vi "ICRA2024测试椭圆分裂.vi"() -> ()   [LabVIEW 2018]
doc: "Demonstrates the use of the Network Streams functions to send LED status to the myRIO target."
uses:
  <vilib>/vision/Contour.llb/IMAQ Contour Curve Extraction.ctl
  <vilib>/ErrorRing/Error Ring.xnode
  <vilib>/vision/NI_Vision_Development_Module.lvlib
panel:
  in  "Search Rect (entire image)":T1={"Left"=200, "Top"=120, "Right"=2000, "Bottom"=1920, "Rotation"=0.0} {"Rotation" format="%.2f"; "Left" scale=0.0..1024.0; "Right" scale=0.0..1024.0}
  out "长度":dbl
  out "备用的椭圆角度":sgl
  in  "打开轨迹":bool
  out "Image 9":T2(plugin-control)
  in  "Search Direction":T3(ring)
  in  "Contour Selection":T4(ring)
  in  "Number of Erosion":i32=10
  in  "椭圆磁场开关":bool=TRUE
  out "Image 7":T2(plugin-control)
  out "Ellipse":T5 {"Center"."Y" format="%.2f"; "Center"."X" format="%.2f"}
  out "Image 5":T2(plugin-control)
  in  "Contour Points Settings":T6={"Overlay?"=FALSE, "Color"=16711680, "Width"=1, "Maintain Width?"=TRUE}
  in  "Contour Equation Settings":T6={"Overlay?"=TRUE, "Color"=3381759, "Width"=1, "Maintain Width?"=TRUE}
  out "ROI Descriptor Out":T7 {"Contours"."Type" items=["No Selection", "Point", "Line", "Rectangle", "Oval", "Polygon", "Freehand Region", "Annulus", "Unused2", "Unused3", "Broken Line", "Freehand Line", "Rotated Rectangle"]}
  in  "Curve Extraction":T8={"Extraction Mode"=0, "Edge Threshold"=75, "Edge Filter Size"=1, "Min Length"=25, "Search Step Size"=15, "Max Endpoint Gap"=10, "Subpixel"=TRUE} {"Extraction Mode" items=["Normal", "Uniform Regions"]; "Edge Filter Size" items=["Fine", "Normal", "Contour Tracing"]; "Max Endpoint Gap" min=0; "Search Step Size" min=1 max=255 step=1; "Min Length" min=0; "Edge Threshold" min=1 max=350 step=1}
  out "Image 4":T2(plugin-control)
  out "Image":T2(plugin-control)
  in  "Acquisition Control::Acquisition Frame Rate":dbl=19.50304412841797 min=1.4211589097976685 max=44.94382095336914
  out "Stopped":bool
  in  "Stop (F) 2":bool caption="Stop (F)"
  out "Objects 2":T9(array[cluster]) {"Aspect Ratio" format="%.2f"; "Orientation" format="%.2f"; "Area" format="%.2f"; "Object Center"."Y" format="%.2f"; "Object Center"."X" format="%.2f"}
  in  "Settings 2":T10={"Objects"=0, "Threshold"=128, "Reject Border"=FALSE, "Fill Holes"=FALSE, "Min Object Size"=TRUE, "Min Size"=20000, "Max Object Size"=FALSE, "Max Size"=100, "Show Search Area"=FALSE, "Show Center"=TRUE, "Show Bounding Box"=TRUE} {"Objects" items=["Bright Objects", "Dark Objects"]; "Threshold" min=1 max=999999999 step=1; "Max Size" min=1 max=999999999 step=1; "Min Size" min=1 max=999999999 step=1}
  in  "Range 2":cluster{"Lower value":sgl, "Upper value":sgl}={"Lower value"=0.0, "Upper value"=230.0} {"Upper value" format="%.2f"; "Lower value" format="%.2f"}
  in  "Pause":bool
  out "Array":dbl[](array[numeric])
  in  "Parameter Settings":T11(tab)=enum."Ribbon Oscillating Field" caption="Field Types"
  in  "fg":dbl
  in  "pg":dbl
  in  "dg":dbl
  in  "Ag":dbl
  in  "AoOF":dbl
  in  "fo":sgl
  in  "do":sgl
  in  "oo":sgl
  in  "po":sgl
  in  "cc":sgl
  in  "pc":sgl
  in  "wc":sgl
  in  "dc":sgl
  in  "Ac":dbl
  in  "pr":sgl
  in  "Ar":dbl=8.0
  in  "wr":sgl=18.0
  in  "dr":sgl
  in  "Dis phase step":dbl
  in  "Dis phase frequency (Hz)":dbl
  in  "Dis tumbling frequency (Hz)":dbl
  in  "Dis strength(mT)":dbl
  in  "Swa strength (mT)":dbl
  in  "Swa frequency (Hz)":dbl
  in  "Swa pitch angle (deg)":dbl
  in  "Swa direction angle (deg)":dbl
  in  "Swa ratio":dbl=1.0
  in  "Pitch Angle (rotating around Constant, deg)":dbl
  in  "Ratio (A/C)":sgl=4.0
  in  "Direction Angle (deg)":sgl
  in  "Pitch Angle (rotating around Origin, deg)":sgl
  in  "Frequency (Hz)":sgl=10.0
  in  "Strength (mT)":dbl=10.0
  in  "Ar 2":dbl=5.0 caption="Ar"
  in  "ratio":sgl=1.0
  in  "运动方向":sgl
  in  "长轴方向":sgl
  in  "wr  2":sgl=8.0
  in  "速度大小":sgl
  out "Angle":dbl
  out "aspect ratio":dbl
  out "时间":i32
  out "Numeric 5":i32
  in  "Stop":bool
  out "error out":errorcluster
  in  "Target IP Address":string="172.22.11.2"
  # "Overview: Magnetic field calculation, and send parameters to myRIO\nInstructions:\n1. Verify the value of Target IP Address. Set Visa resource name.\n2. Ensure RT Main.vi is already running. \n3. Run this VI. Set parameters of magnetic field."
  # "Strength (mT)"
  # "Pitch Angle (deg)"
  # "Direction Angle (deg)"
  # "Frequency (Hz)"
  # "Strength (mT)"
  # "Oscilation Frequency (Hz)"
  # "Oscilation Angle (deg)"
  # "Pitch Angle (deg)"
  # "Direction Angle (deg)"
  # "Strength (mT)"
  # "Frequency (Hz)"
  # "Pitch Angle (deg)"
  # "Direction Angle (deg)"
  # "Conical Angle (deg)"
  # "Strength (mT)"
  # "Frequency (Hz)"
  # "Pitch Angle (deg)"
  # "Direction Angle (deg)"
  # "Strength (mT)"
  # "Tumbling Frequency (Hz)"
  # "Phase Frequency (Hz)"
  # "Phase Step"
  # "Strength (mT)"
  # "Frequency (Hz)"
  # "Pitch Angle (deg)"
  # "Direction Angle (deg)"
  # "Ratio"
  # "Strength (mT)"
  # "Frequency (Hz)"
  # "Ratio (A/C)"
  # "Direction Angle (deg)"
  # "Pitch Angle (rotating around Origin, deg)"
  # "Pitch Angle (rotating around Constant, deg)"
  # "Strength (mT)"
  # "Frequency (Hz)"
  # "Pitch Angle  (deg)"
  # "longaxis"
  # "Direction Angle (deg)"
  # "ratio (l/s)"
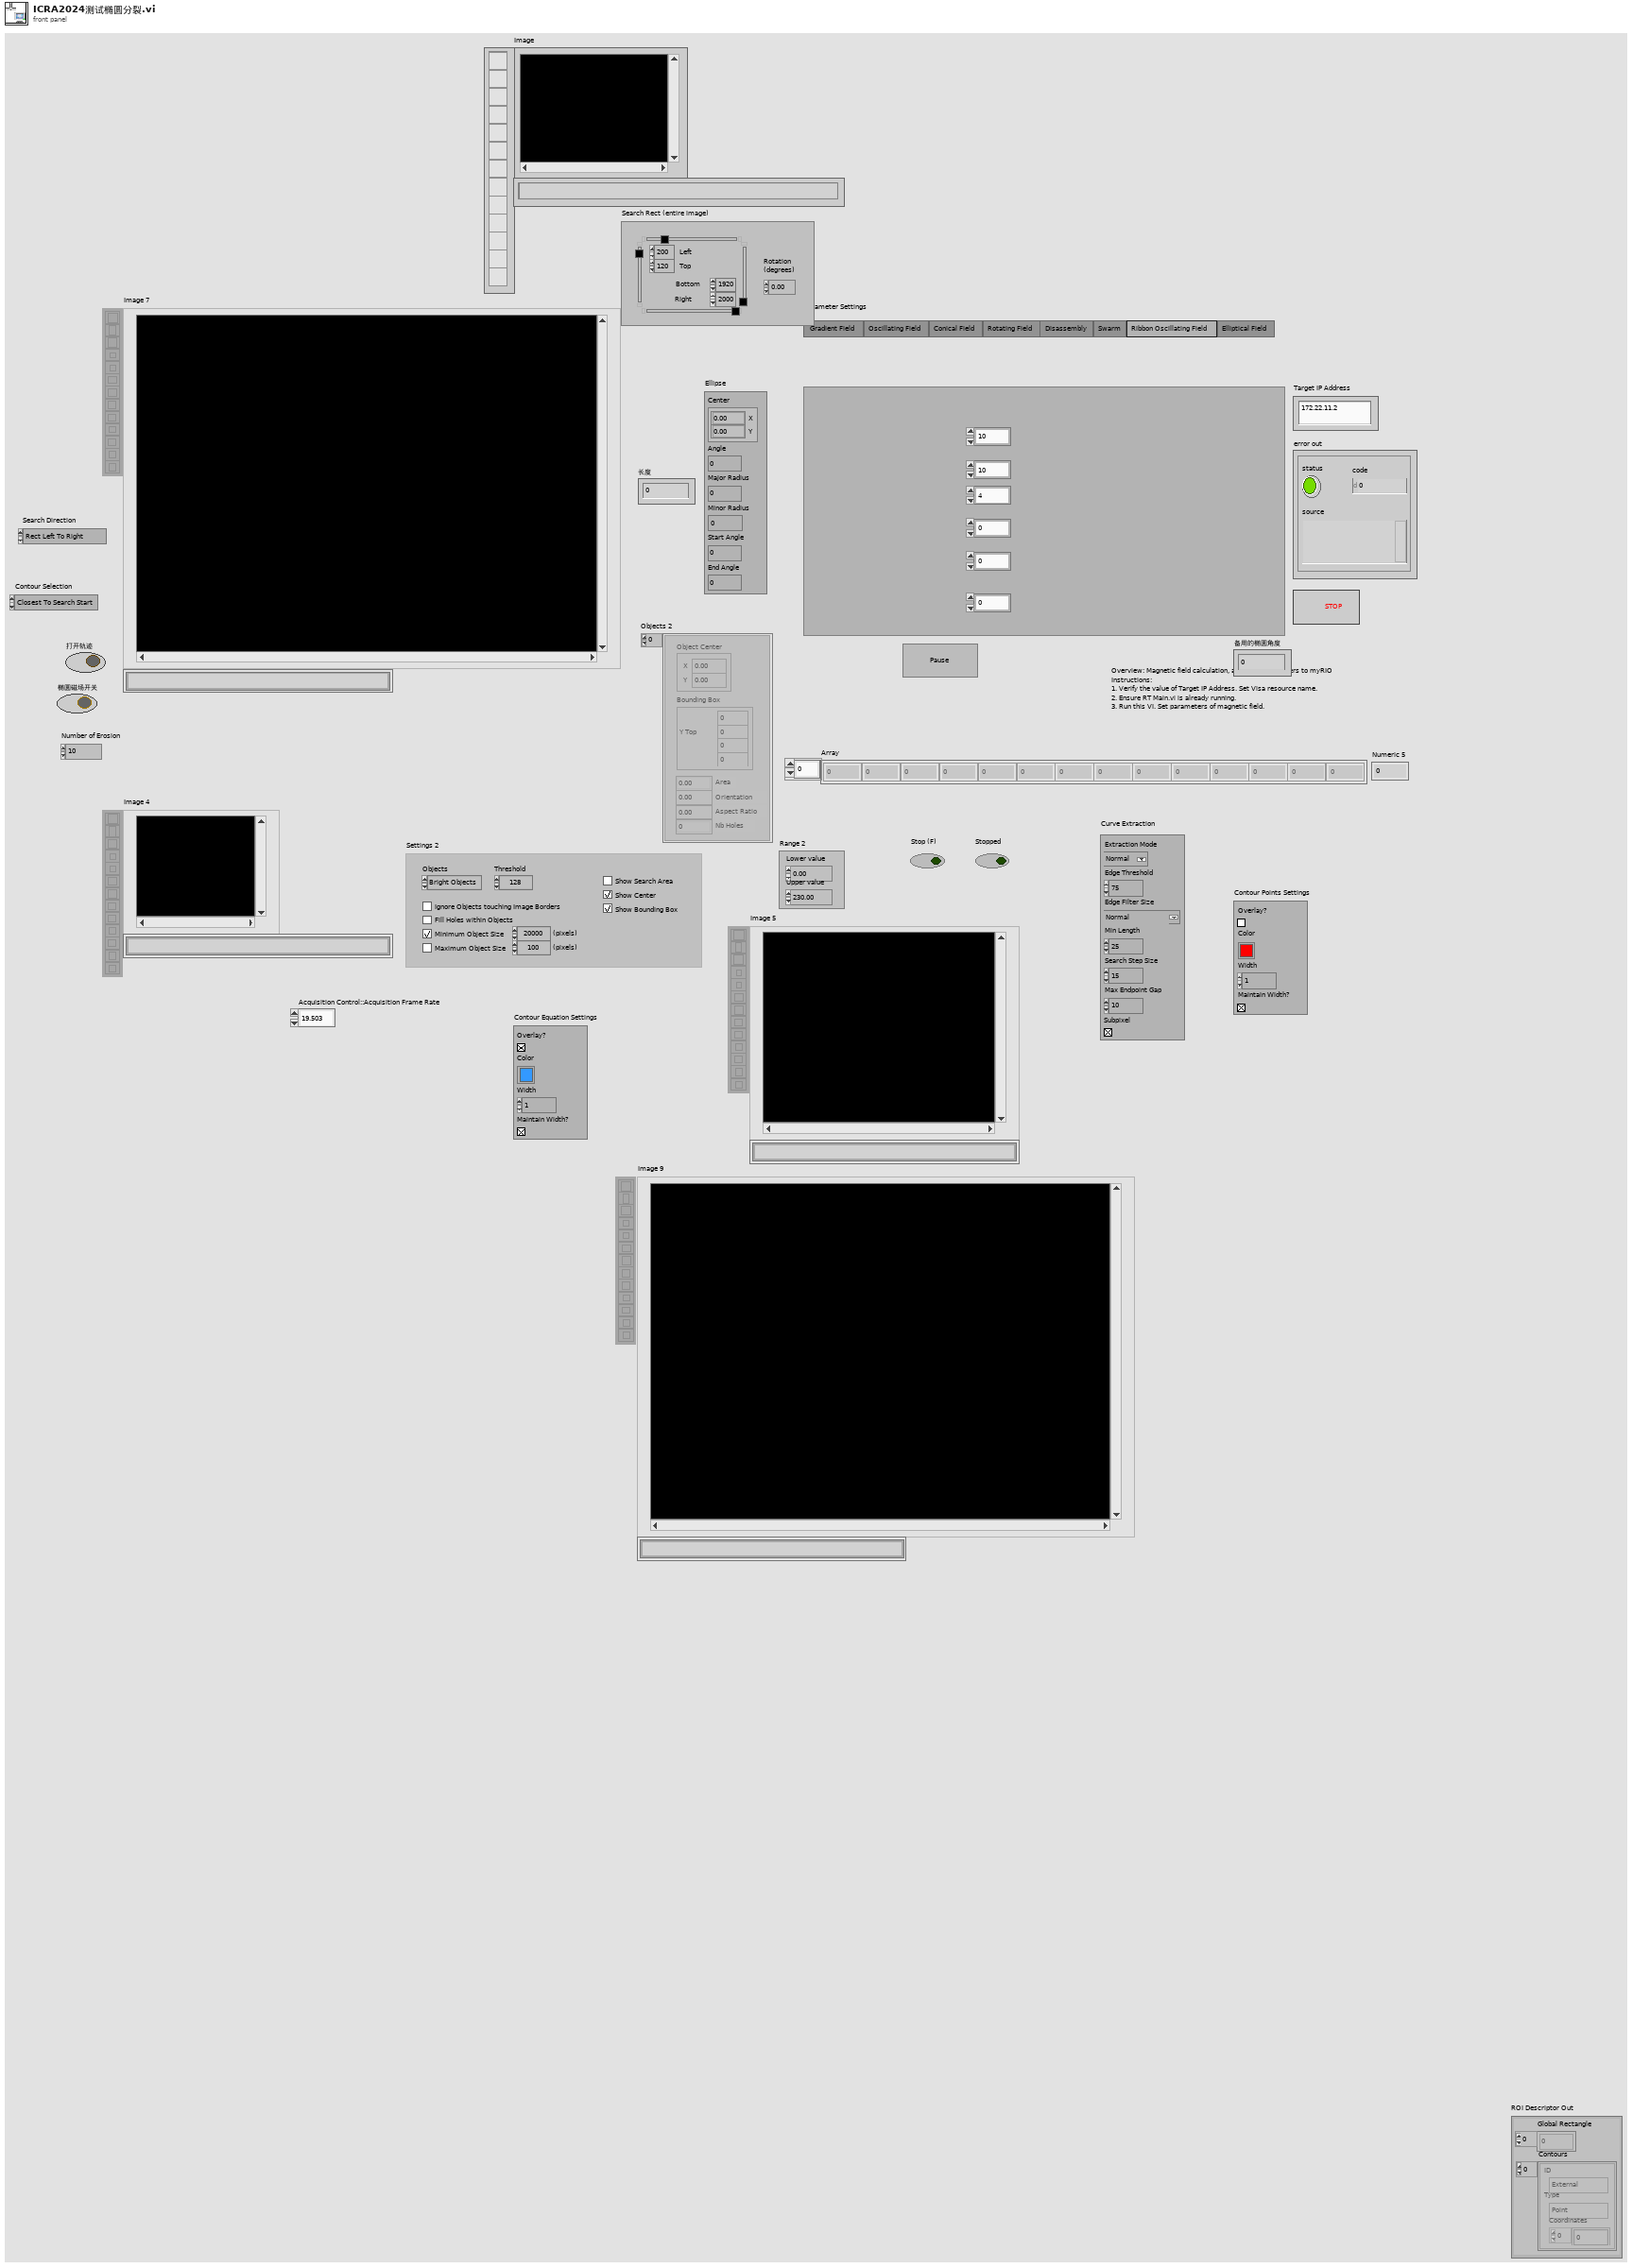
[diagram p1: front panel]
types:
  T1 = typedef "IMAQ Rectangle" = cluster{"Left":i32, "Top":i32, "Right":i32, "Bottom":i32, "Rotation":dbl}
  T2 = typedef "IMAQ Image.ctl" = refnum<image>
  T3 = enum16{"Rect Left To Right", "Rect Right To Left", "Rect Top To Bottom", "Rect Bottom To Top", "Annulus Inner To Outer", "Annulus Outer To Inner", "Annulus Start Angle To End Angle", "Annulus End Angle To Start Angle"}
  T4 = enum16{"Closest To Search Start", "Maximum Length", "Strongest Mean Gradient Change"}
  T5 = cluster{"Center":cluster{"X":sgl, "Y":sgl}, "Angle":dbl, "Major Radius":dbl, "Minor Radius":dbl, "Start Angle":dbl, "End Angle":dbl}
  T6 = cluster{"Overlay?":bool, "Color":u32, "Width":u32, "Maintain Width?":bool}
  T7 = typedef "ROI Descriptor" = cluster{"Global Rectangle":i32[], "Contours":cluster{"ID":enum32{"External", "Internal"}, "Type":u32, "Coordinates":i32[]}[]}
  T8 = typedef "IMAQ Contour Curve Extraction.ctl" = cluster{"Extraction Mode":u32, "Edge Threshold":i32, "Edge Filter Size":u32, "Min Length":i32, "Search Step Size":i32, "Max Endpoint Gap":i32, "Subpixel":bool}
  T9 = cluster{"Object Center":cluster{"X":sgl, "Y":sgl}, "Bounding Box":cluster{"X Left":i32, "Y Top":i32, "X Right":i32, "Y Bottom":i32}, "Area":sgl, "Orientation":sgl, "Aspect Ratio":sgl, "Nb Holes":i32}[]
  T10 = cluster{"Objects":u16, "Threshold":i32, "Reject Border":bool, "Fill Holes":bool, "Min Object Size":bool, "Min Size":i32, "Max Object Size":bool, "Max Size":i32, "Show Search Area":bool, "Show Center":bool, "Show Bounding Box":bool}
  T11 = enum32{"Gradient Field ", "Oscillating Field", "Conical Field", "Rotating Field", "Disassembly", "Swarm", "Ribbon Oscillating Field", "Elliptical Field"}
  T12 = enum32{"AutoM", "Close", "Dilate", "Erode", "Gradient", "Gradient in", "Gradient out", "HitMiss", "Open", "PClose", "POpen", "Thick", "Thin"}
  T13 = typedef "Image Type" = u32
  T14 = cluster{"Objects[0]":cluster{"Object Center":cluster{"X":sgl, "Y":sgl}, "Bounding Box":cluster{"X Left":i32, "Y Top":i32, "X Right":i32, "Y Bottom":i32}, "Area":sgl, "Orientation":sgl, "Aspect Ratio":sgl, "Nb Holes":i32}, "Objects[1]":cluster{"Object Center":cluster{"X":sgl, "Y":sgl}, "Bounding Box":cluster{"X Left":i32, "Y Top":i32, "X Right":i32, "Y Bottom":i32}, "Area":sgl, "Orientation":sgl, "Aspect Ratio":sgl, "Nb Holes":i32}, "Objects[2]":cluster{"Object Center":cluster{"X":sgl, "Y":sgl}, "Bounding Box":cluster{"X Left":i32, "Y Top":i32, "X Right":i32, "Y Bottom":i32}, "Area":sgl, "Orientation":sgl, "Aspect Ratio":sgl, "Nb Holes":i32}, "Objects[3]":cluster{"Object Center":cluster{"X":sgl, "Y":sgl}, "Bounding Box":cluster{"X Left":i32, "Y Top":i32, "X Right":i32, "Y Bottom":i32}, "Area":sgl, "Orientation":sgl, "Aspect Ratio":sgl, "Nb Holes":i32}, "Objects[4]":cluster{"Object Center":cluster{"X":sgl, "Y":sgl}, "Bounding Box":cluster{"X Left":i32, "Y Top":i32, "X Right":i32, "Y Bottom":i32}, "Area":sgl, "Orientation":sgl, "Aspect Ratio":sgl, "Nb Holes":i32}, "Objects[5]":cluster{"Object Center":cluster{"X":sgl, "Y":sgl}, "Bounding Box":cluster{"X Left":i32, "Y Top":i32, "X Right":i32, "Y Bottom":i32}, "Area":sgl, "Orientation":sgl, "Aspect Ratio":sgl, "Nb Holes":i32}, "Objects[6]":cluster{"Object Center":cluster{"X":sgl, "Y":sgl}, "Bounding Box":cluster{"X Left":i32, "Y Top":i32, "X Right":i32, "Y Bottom":i32}, "Area":sgl, "Orientation":sgl, "Aspect Ratio":sgl, "Nb Holes":i32}, "Objects[7]":cluster{"Object Center":cluster{"X":sgl, "Y":sgl}, "Bounding Box":cluster{"X Left":i32, "Y Top":i32, "X Right":i32, "Y Bottom":i32}, "Area":sgl, "Orientation":sgl, "Aspect Ratio":sgl, "Nb Holes":i32}, "Objects[8]":cluster{"Object Center":cluster{"X":sgl, "Y":sgl}, "Bounding Box":cluster{"X Left":i32, "Y Top":i32, "X Right":i32, "Y Bottom":i32}, "Area":sgl, "Orientation":sgl, "Aspect Ratio":sgl, "Nb Holes":i32}}
  T15 = cluster{"Object Center":cluster{"X":sgl, "Y":sgl}, "Bounding Box":cluster{"X Left":i32, "Y Top":i32, "X Right":i32, "Y Bottom":i32}, "Area":sgl, "Orientation":sgl, "Aspect Ratio":sgl, "Nb Holes":i32}
  T16 = cluster{"X Left":i32, "Y Top":i32, "X Right":i32, "Y Bottom":i32}
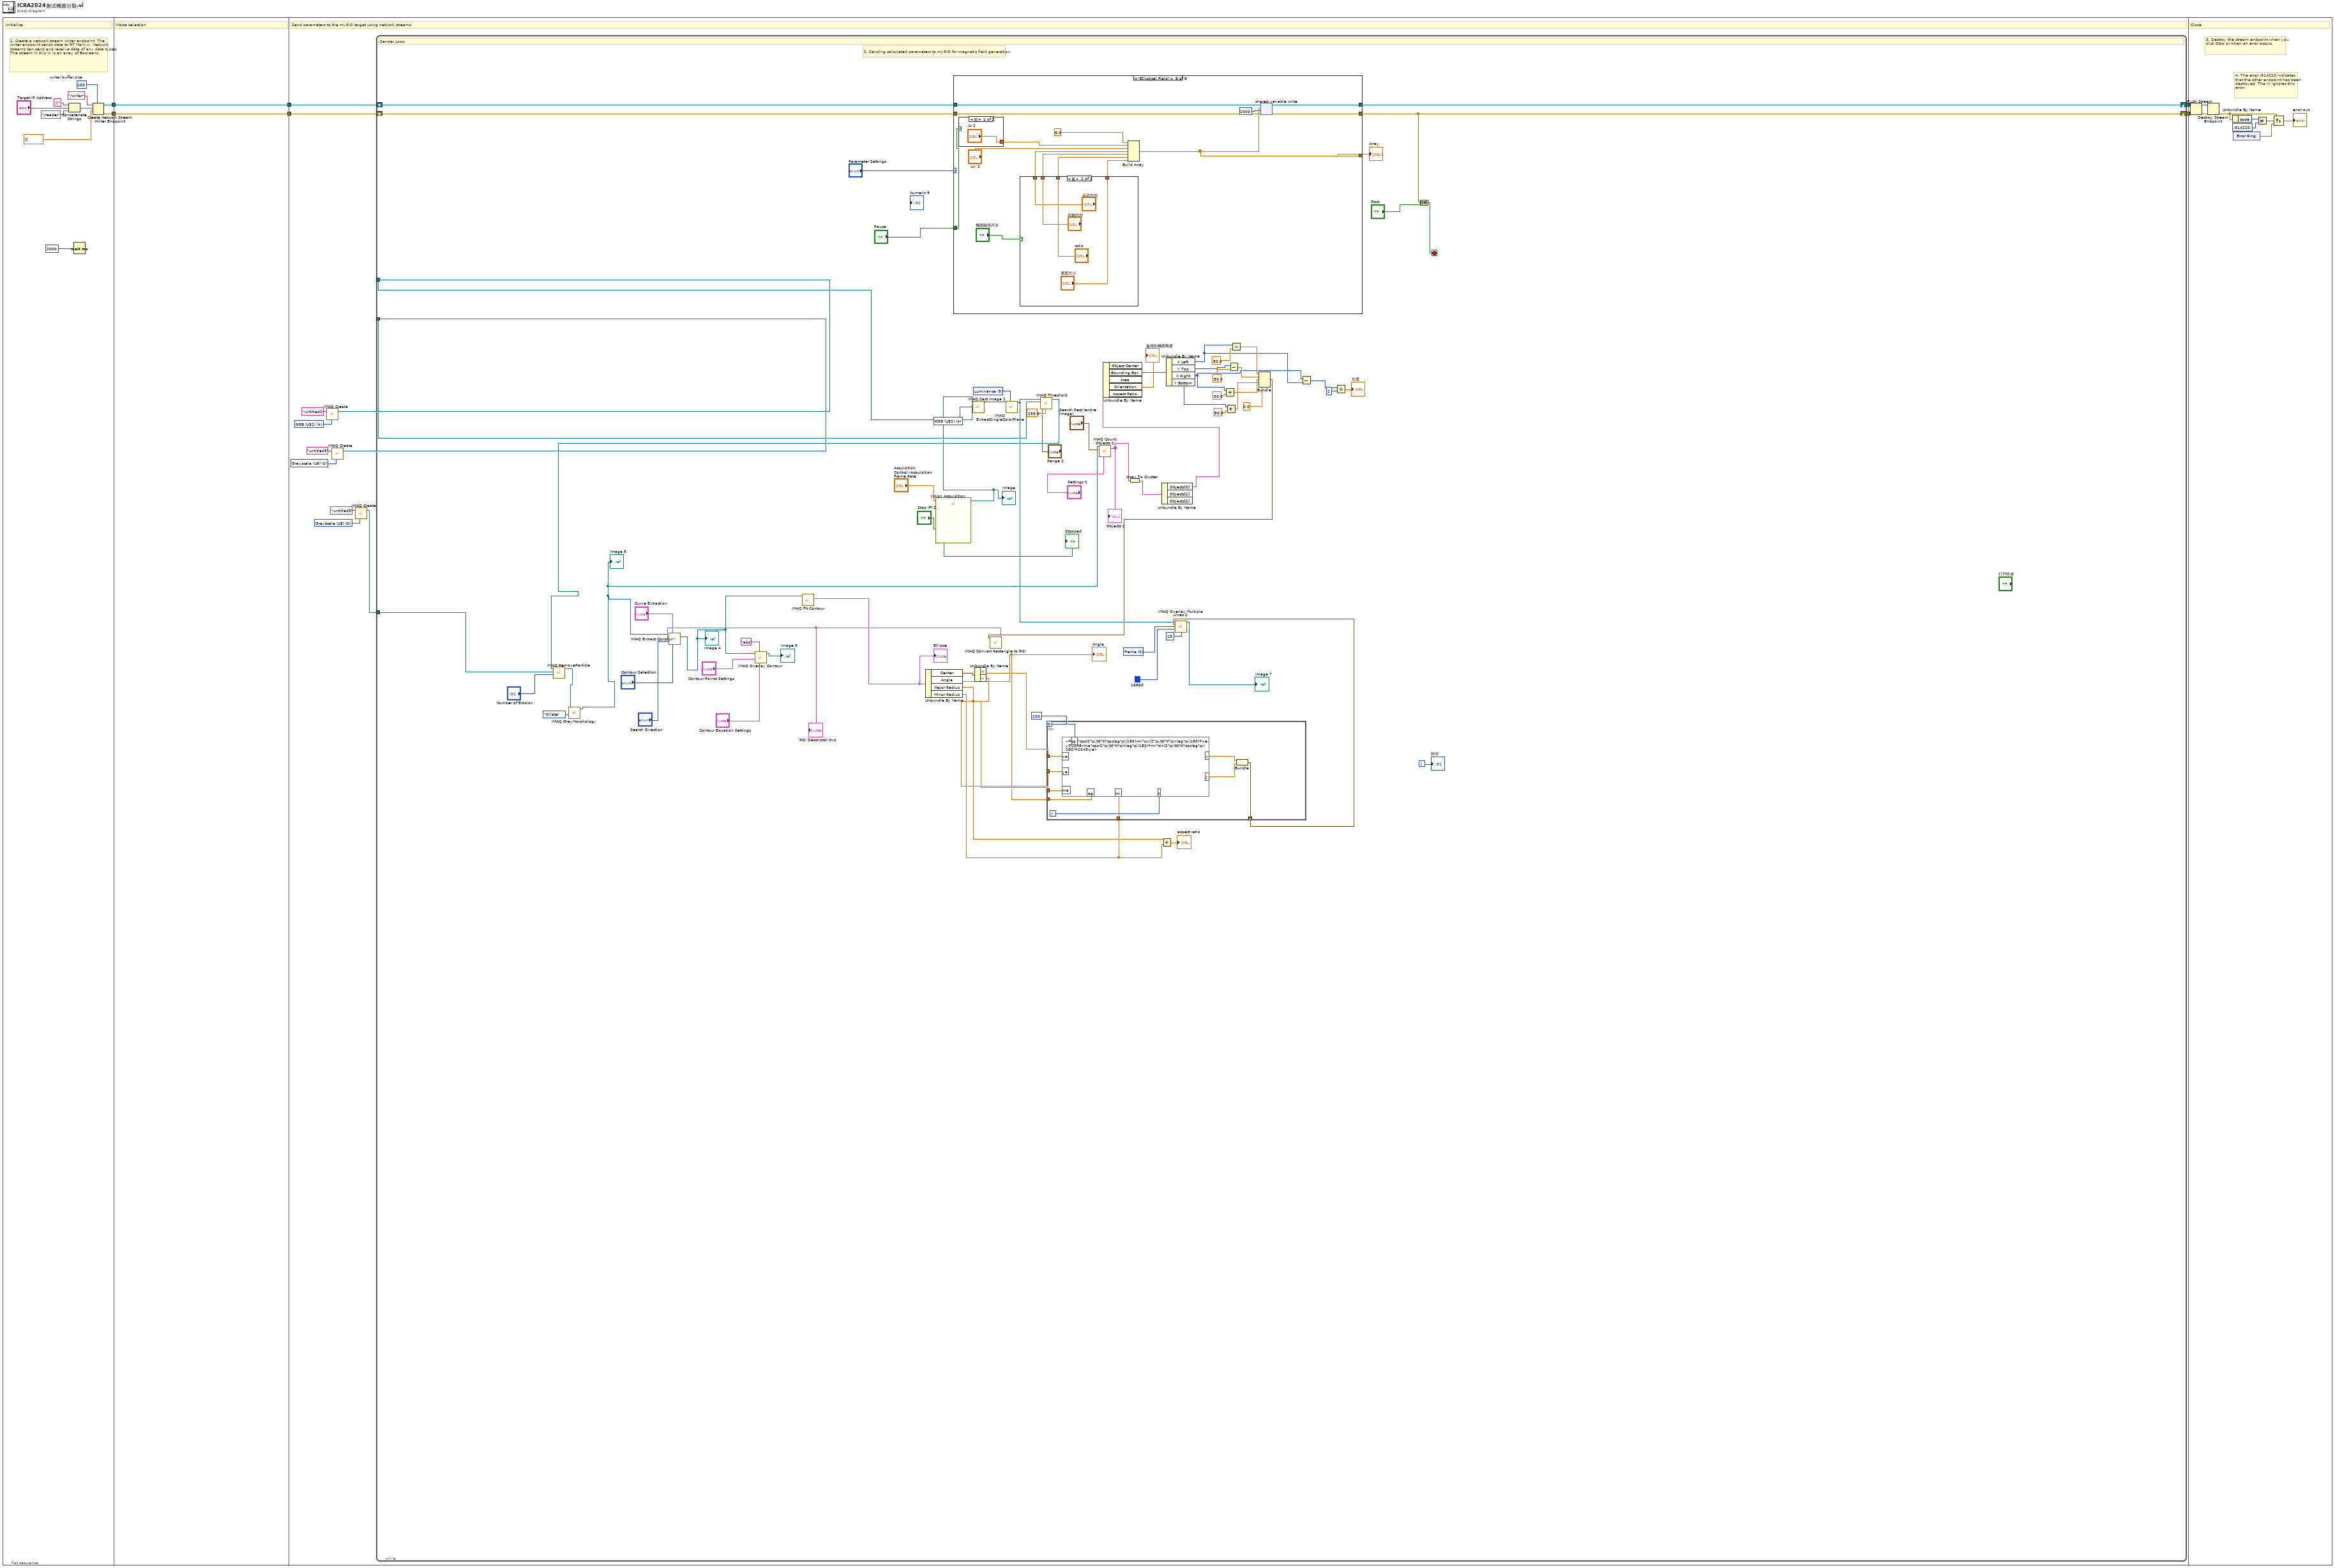
[diagram p0: block diagram]
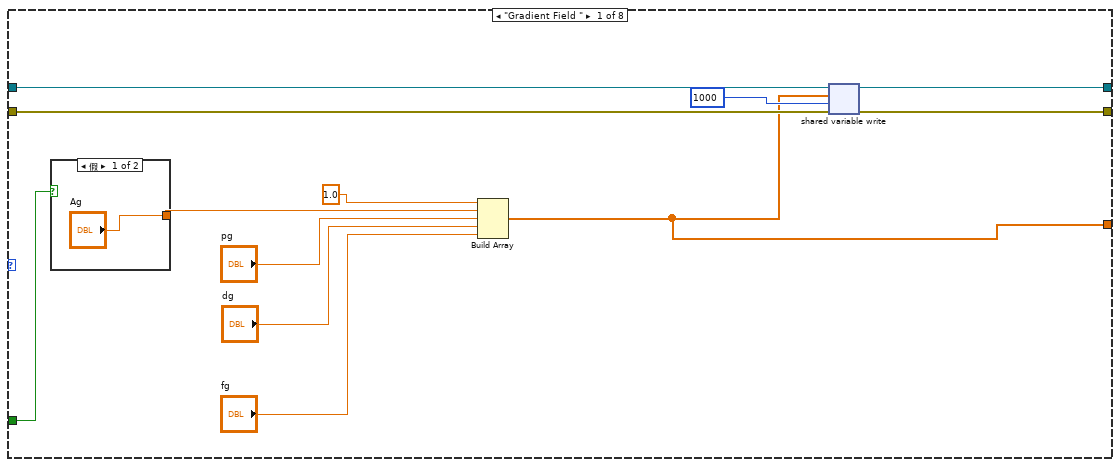
[diagram p2: hidden frame]
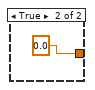
[diagram p3: hidden frame]
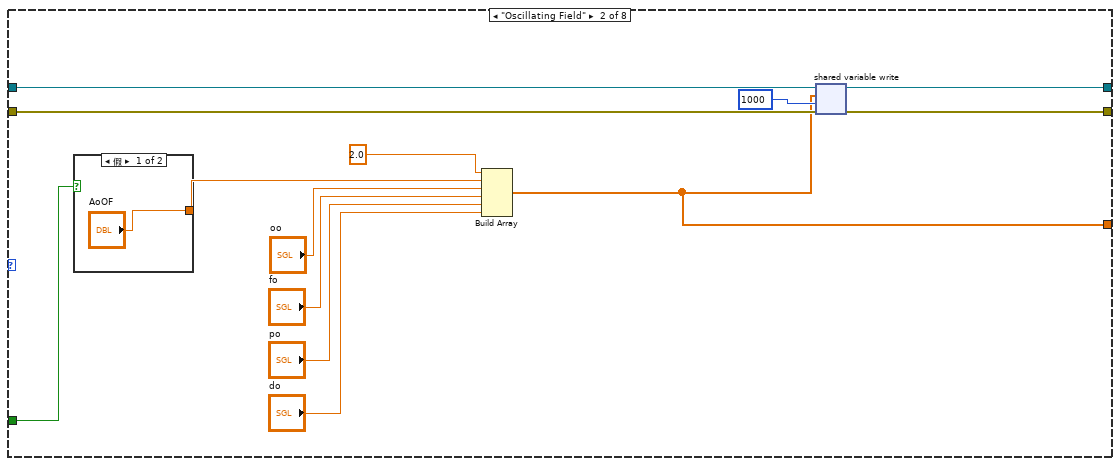
[diagram p4: hidden frame]
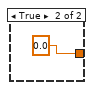
[diagram p5: hidden frame]
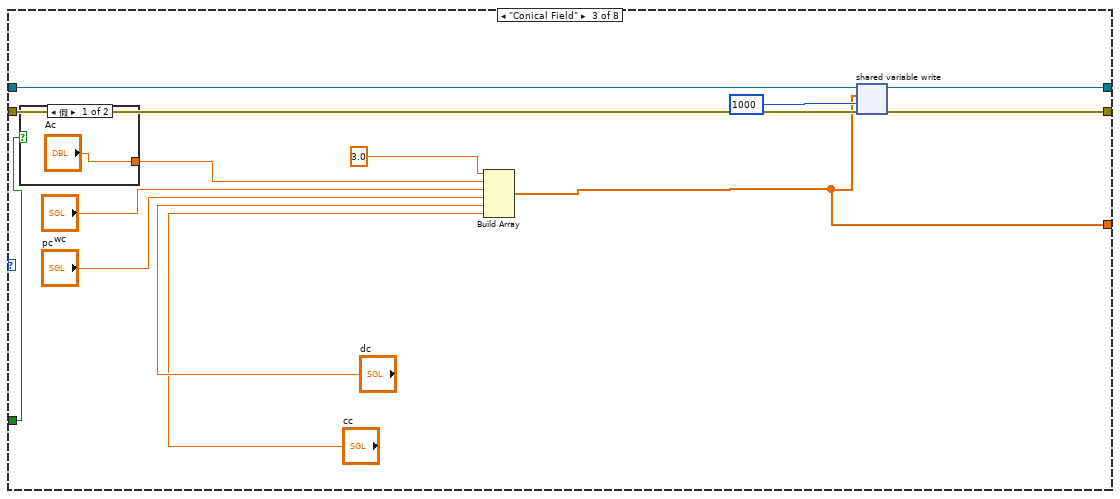
[diagram p6: hidden frame]
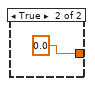
[diagram p7: hidden frame]
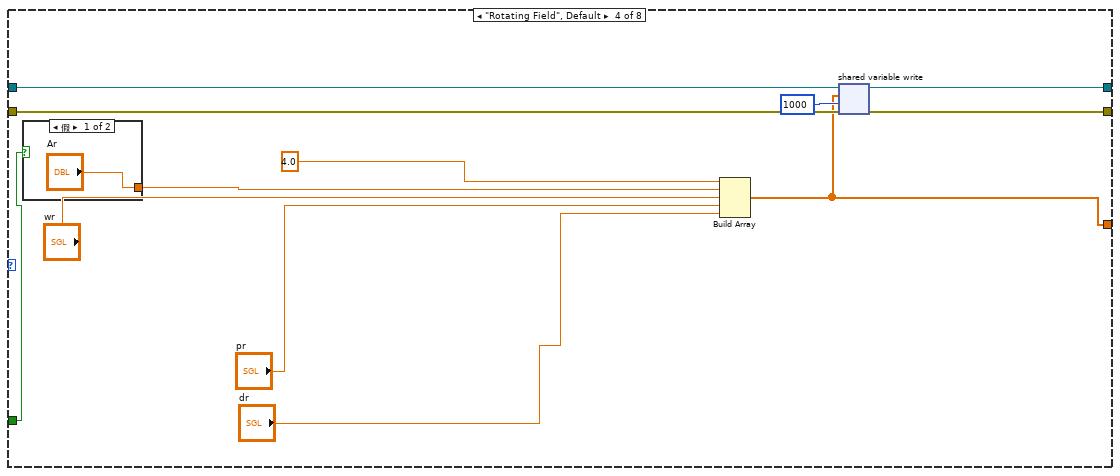
[diagram p8: hidden frame]
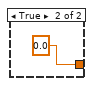
[diagram p9: hidden frame]
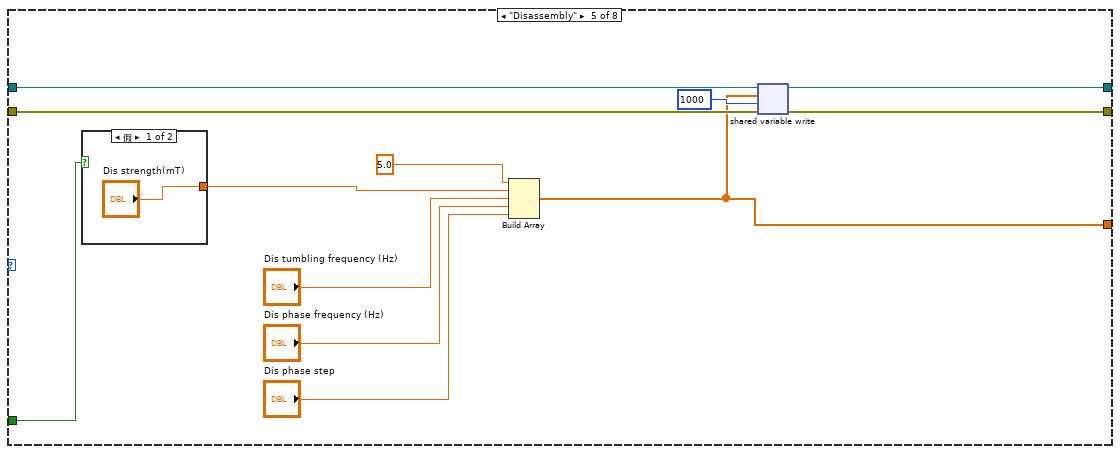
[diagram p10: hidden frame]
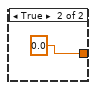
[diagram p11: hidden frame]
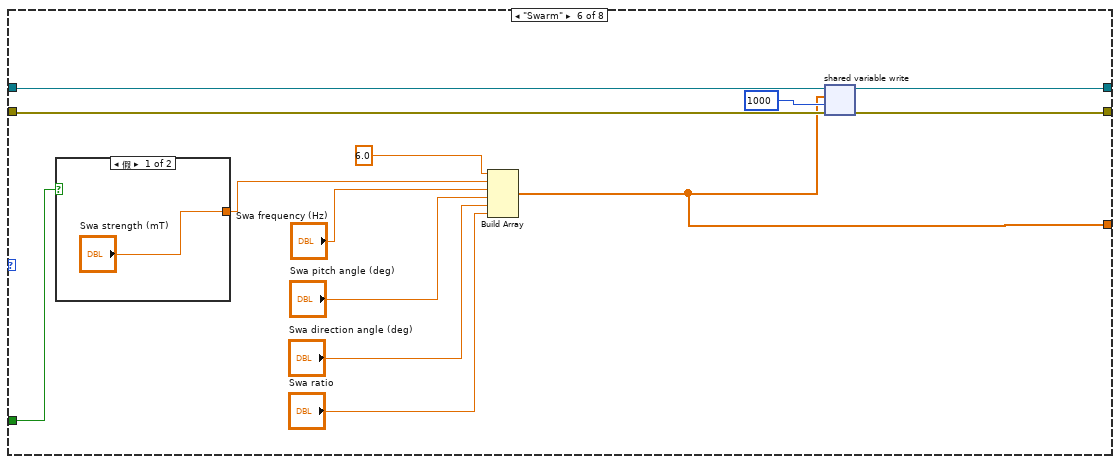
[diagram p12: hidden frame]
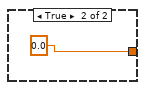
[diagram p13: hidden frame]
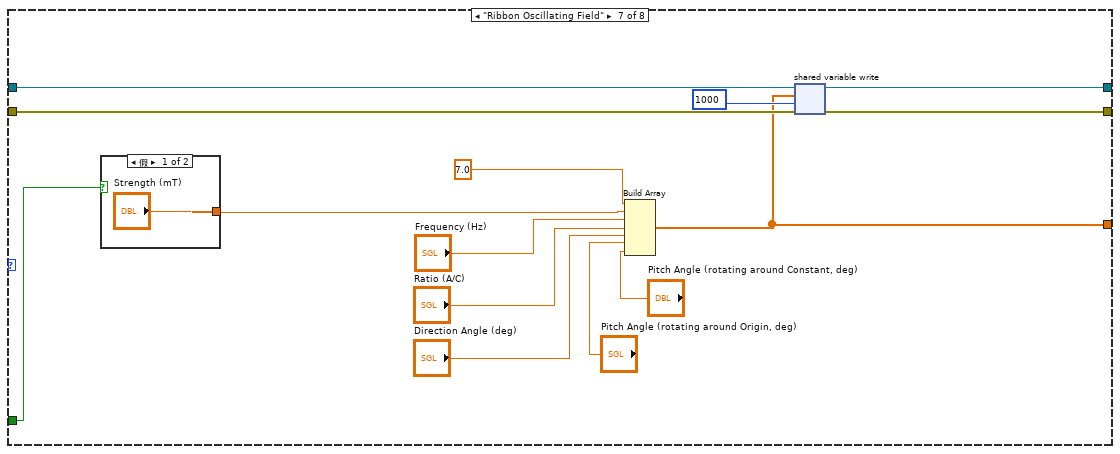
[diagram p14: hidden frame]
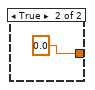
[diagram p15: hidden frame]
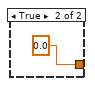
[diagram p17: hidden frame]
diagram:
  n1 = flat-sequence {
    tunnel: [w11] -> w2
    tunnel: [w10] -> w1
    tunnel: [w18] -> w4
    tunnel: [w17] -> w3
    tunnel: w1 -> [w17]
    tunnel: w2 -> [w18]
    tunnel: [w29] -> w6
    tunnel: w4 -> [w31]
    tunnel: [w28] -> w5
    tunnel: w3 -> [w30]
    tunnel: w6 -> [w250]
    tunnel: w5 -> [w247]
    frame #0 {
      w9 = 100  # writer buffer size
      # "1. Create a network stream writer endpoint. The writer endpoint sends data to RT Main.vi. Network streams can send and receive data of any data types. The stream in this VI is an array of Booleans."
      # "Initialize"
      n2 = Concatenate Strings("//", "Target IP Address", "/reader") -> (w16:string)
      n3 = Wait (ms)(milliseconds to wait=2000) -> ()  [unwired: 1 out]
      n4 = Create Network Stream Writer Endpoint(7:w9, 9:dbl[] [], 10:w16, 11:"/writer" ("reader name")) -> (0:w10:errorcluster, 3:w11:refnum<k21>)  [unwired: 3 in]
    }
    frame #1 {
      # "Mode selection"
    }
    frame #2 {
      w20 = T13 0 items=["Grayscale (U8)", "Grayscale (I16)", "Grayscale (SGL)", "Complex (CSG)", "RGB (U32)", "HSL (U32)", "RGB (U64)", "Grayscale (U16)"] ("Image Type")
      w24 = T13 0 items=["Grayscale (U8)", "Grayscale (I16)", "Grayscale (SGL)", "Complex (CSG)", "RGB (U32)", "HSL (U32)", "RGB (U64)", "Grayscale (U16)"] ("Image Type")
      w26 = T13 4 items=["Grayscale (U8)", "Grayscale (I16)", "Grayscale (SGL)", "Complex (CSG)", "RGB (U32)", "HSL (U32)", "RGB (U64)", "Grayscale (U16)"] ("Image Type")
      # "Send parameters to the myRIO target using network streams"
      n5 = call "IMAQ Create"("Image Name"="untitled2", "Image Type"=w26) -> ("New Image"=w23:T2)  [unwired: 3 in, 1 out]
      n6 = call "IMAQ Create"("Image Name"="untitled3", "Image Type"=w24) -> ("New Image"=w22:T2)  [unwired: 3 in, 1 out]
      n7 = call "IMAQ Create"("Image Name"="untitled3", "Image Type"=w20) -> ("New Image"=w19:T2)  [unwired: 3 in, 1 out]
      n8 = while {
        shift-right: [w102] -> w28
        shift-left: w30 -> [w104]
        shift-right: [w103] -> w29
        shift-left: w31 -> [w105]
        tunnel: w22 -> [w93]
        tunnel: w23 -> [w88]
        tunnel: w19 -> [w56]
        i -> [w39]
        stop <- w92 stop-if-true
        w75 = u32 0 items=["Frame", "Fill"] ("Drawing Mode (Frame)")
        w87 = T13 4 items=["Grayscale (U8)", "Grayscale (I16)", "Grayscale (SGL)", "Complex (CSG)", "RGB (U32)", "HSL (U32)", "RGB (U64)", "Grayscale (U16)"] ("Image Type")
        w98 = 5 items=["Red", "Green", "Blue", "Hue", "Saturation", "Luminance", "Value", "Intensity"] ("Color Plane")
        # "2. Sending calculated parameters to myRIO for magnetic field generation."
        # "Sender Loop"
        n9 = call "Vision Acquisition"("Acquisition Control::Acquisition Frame Rate"="Acquisition Control::Acquisition Frame Rate", "Stop (F)"="Stop (F) 2") -> ("Image Out"=w86:T2, "Stopped"=→"Stopped":bool)  [unwired: 23 in, 1 out]
        "Image" <- w86
        n10 = case shown="\"Elliptical Field\"" "Parameter Settings" {
          tunnel: w105 -> [w127 w142 w157 w171 w185 w199 w217 w233]
          tunnel: w104 -> [w124 w141 w156 w170 w183 w198 w215 w232]
          tunnel: [w126 w140 w154 w169 w184 w197 w216 w231] -> w103
          tunnel: [w125 w139 w155 w168 w182 w196 w214 w230] -> w102
          tunnel: [w120 w133 w148 w163 w176 w191 w212 w225] -> w101
          tunnel: "Pause" -> [w118 w131 w146 w161 w175 w190 w207 w223]
          frame "Gradient Field " {
            n11 = case shown="假" w118 {
              tunnel: ["Ag" 0.0] -> w119
              frame False {
              }
              frame True {
              }
            }
            n12 = Build Array(1.0, w119, "pg", "dg", "fg") -> (w120:dbl[])
            n13 = shared-variable-write(w127, w124, w120, 1000 ("timeout ms (-1)")) -> (w126:refnum<k21>, w125:errorcluster)  [unwired: 1 out]
          }
          frame "Oscillating Field" {
            n14 = case shown="假" w131 {
              tunnel: ["AoOF" 0.0] -> w132
              frame False {
              }
              frame True {
              }
            }
            n15 = Build Array(2.0, w132, "oo", "fo", "po", "do") -> (w133:dbl[])
            n16 = shared-variable-write(w142, w141, w133, 1000 ("timeout ms (-1)")) -> (w140:refnum<k21>, w139:errorcluster)  [unwired: 1 out]
          }
          frame "Conical Field" {
            # "FG"
            n17 = case shown="假" w146 {
              tunnel: ["Ac" 0.0] -> w147
              frame False {
              }
              frame True {
              }
            }
            n18 = Build Array(3.0, w147, "wc", "pc", "dc", "cc") -> (w148:dbl[])
            n19 = shared-variable-write(w157, w156, w148, 1000 ("timeout ms (-1)")) -> (w154:refnum<k21>, w155:errorcluster)  [unwired: 1 out]
          }
          frame "Rotating Field", Default {
            n20 = case shown="假" w161 {
              tunnel: ["Ar" 0.0] -> w162
              frame False {
              }
              frame True {
              }
            }
            n21 = Build Array(4.0, w162, "wr", "pr", "dr") -> (w163:dbl[])
            n22 = shared-variable-write(w171, w170, w163, 1000 ("timeout ms (-1)")) -> (w169:refnum<k21>, w168:errorcluster)  [unwired: 1 out]
          }
          frame "Disassembly" {
            n23 = case shown="假" w175 {
              tunnel: ["Dis strength(mT)" 0.0] -> w180
              frame False {
              }
              frame True {
              }
            }
            n24 = Build Array(5.0, w180, "Dis tumbling frequency (Hz)", "Dis phase frequency (Hz)", "Dis phase step") -> (w176:dbl[])
            n25 = shared-variable-write(w185, w183, w176, 1000 ("timeout ms (-1)")) -> (w184:refnum<k21>, w182:errorcluster)  [unwired: 1 out]
          }
          frame "Swarm" {
            n26 = case shown="假" w190 {
              tunnel: ["Swa strength (mT)" 0.0] -> w189
              frame False {
              }
              frame True {
              }
            }
            n27 = Build Array(6.0, w189, "Swa frequency (Hz)", "Swa pitch angle (deg)", "Swa direction angle (deg)", "Swa ratio") -> (w191:dbl[])
            n28 = shared-variable-write(w199, w198, w191, 1000 ("timeout ms (-1)")) -> (w197:refnum<k21>, w196:errorcluster)  [unwired: 1 out]
          }
          frame "Ribbon Oscillating Field" {
            n29 = case shown="假" w207 {
              tunnel: ["Strength (mT)" 0.0] -> w206
              frame False {
              }
              frame True {
              }
            }
            n30 = Build Array(7.0, w206, "Frequency (Hz)", "Ratio (A/C)", "Direction Angle (deg)", "Pitch Angle (rotating around Origin, deg)", "Pitch Angle (rotating around Constant, deg)") -> (w212:dbl[])
            n31 = shared-variable-write(w217, w215, w212, 1000 ("timeout ms (-1)")) -> (w216:refnum<k21>, w214:errorcluster)  [unwired: 1 out]
          }
          frame "Elliptical Field" {
            n32 = case shown="假" w223 {
              tunnel: ["Ar 2" 0.0] -> w224
              frame False {
              }
              frame True {
              }
            }
            n33 = case shown="真" "椭圆磁场开关" {
              tunnel: [_ "运动方向"] -> w228
              tunnel: [_ "长轴方向"] -> w227
              tunnel: [_ "ratio"] -> w222
              tunnel: [_ "速度大小"] -> w221
              frame False {
              }
              frame True {
              }
            }
            n34 = Build Array(8.0, w224, "wr  2", w228, w227, w222, w221) -> (w225:dbl[])
            n35 = shared-variable-write(w233, w232, w225, 1000 ("timeout ms (-1)")) -> (w231:refnum<k21>, w230:errorcluster)  [unwired: 1 out]
          }
        }
        "Array" <- w101
        n36 = call "IMAQ Cast Image 2"("Image Src"=w86, "Image Dst"=w88, "Image Type"=w87) -> ("Image Dst Out"=w89:T2)  [unwired: 11 in, 1 out]
        n37 = call "IMAQ ExtractSingleColorPlane"("Color Plane"=w98, "Image Src"=w89) -> ("Image Dst Out"=w48:T2)  [unwired: 8 in, 1 out]
        n38 = call "IMAQ Threshold"("Replace Value"=sgl 255.0, "Range"="Range 2", "Image Dst"=w93, "Image Src"=w48) -> ("Image Dst Out"=w57:T2)  [unwired: 6 in, 1 out]
        n39 = call "IMAQ RemoveParticle"("Number of Erosion"="Number of Erosion", "Image Dst"=w56, "Image Src"=w57) -> ("Image Dst Out"=w52:T2)  [unwired: 7 in, 1 out]
        n40 = call "IMAQ GrayMorphology"("Operation"=T12."Dilate", "Image Src"=w52) -> ("Image Dst Out"=w49:T2)  [unwired: 8 in, 1 out]
        "Image 5" <- w49
        n41 = call "IMAQ Count Objects 2"("Settings"="Settings 2", "Search Rect (entire image)"="Search Rect (entire image)", "Image"=w49) -> ("Objects"=w94:T9)  [unwired: 4 in, 4 out]
        "Objects 2" <- w94
        n42 = Array To Cluster(array=w94) -> (cluster=w59:T14)
        n43 = Unbundle By Name(w59) -> ("Objects[0]"=w58:T15)  [unwired: 2 out]
        n44 = Unbundle By Name(w58) -> ("Bounding Box"=w74:T16, "Orientation"=→"备用的椭圆角度":sgl)  [unwired: 3 out]
        n45 = Unbundle By Name(w74) -> ("X Left"=w36:i32, "Y Top"=w69:i32, "X Right"=w37:i32, "Y Bottom"=w68:i32)
        n46 = Add(x=w37, y=50.0) -> (x+y=w65:dbl)
        n47 = Add(x=w68, y=50.0) -> (x+y=w64:dbl)
        n48 = Subtract(x=w69, y=50.0) -> (x-y=w66:dbl)
        n49 = Subtract(x=w36, y=50.0) -> (x-y=w67:dbl)
        n50 = Bundle(w67, w66, w65, w64, 0.0) -> (w62:cluster{dbl, dbl, dbl, dbl, dbl})  [unwired: 1 in]
        n51 = call "IMAQ Convert Rectangle to ROI"("Rectangle"=w62) -> ("ROI Descriptor"=w61:T7)  [unwired: 8 in, 1 out]
        "ROI Descriptor Out" <- w61
        n52 = call "IMAQ Extract Contour"("Source Image"=w49, "Curve Extraction"="Curve Extraction", "ROI Descriptor"=w61, "Search Direction"="Search Direction", "Contour Selection"="Contour Selection") -> ("Contour Image Out"=w81:T2)  [unwired: 6 in, 4 out]
        "Image 4" <- w81
        n53 = call "IMAQ Overlay Contour"("Contour Equation Settings"="Contour Equation Settings", "Group"="abc", "Contour Points Settings"="Contour Points Settings", "Image"=w81) -> ("Image Out"=→"Image 9":T2)  [unwired: 6 in, 1 out]
        n54 = call-poly "IMAQ Fit Contour"("Contour Image"=w81) -> ("Ellipse"=w79:T5)  [unwired: 8 in, 2 out]
        "Ellipse" <- w79
        n55 = Unbundle By Name(w79) -> ("Center"=w80:cluster{"X":sgl, "Y":sgl}, "Angle"=w43:dbl, "Major Radius"=w46:dbl, "Minor Radius"=w47:dbl)
        "Angle" <- w43
        n56 = Unbundle By Name(w80) -> ("X"=w45:sgl, "Y"=w44:sgl)
        n57 = for {
          N: 200 -> [w112]
          tunnel: [w113] -> w60 mode=indexing
          tunnel: w45 -> [w111]
          tunnel: w44 -> [w110]
          tunnel: w46 -> [w109]
          tunnel: w43 -> [w108]
          tunnel: w47 -> [w107]
          i -> [w114]
          n58 = formula code="x=ma*cos(2*pi/t0*t)*cos(ag*pi/180)-mi*sin(2*pi/t0*t)*sin(ag*pi/180)+xe;\ny=2048-(ma*cos(2*pi/t0*t)*sin(ag*pi/180)+mi*sin(2*pi/t0*t)*cos(ag*pi/180)+2048-ye);"("xe"=w111, "ye"=w110, "ma"=w109, "ag"=w108, "mi"=w107, "t"=w114, "t0"=w112) -> ("x"=w116:dbl, "y"=w115:dbl)
          n59 = Bundle("x"=w116, "y"=w115) -> (w113:cluster{"x":dbl, "y":dbl})  [unwired: 1 in]
        }
        n60 = Divide(x=w46, y=w47) -> (x/y=→"aspect ratio":dbl)
        n61 = call "IMAQ Overlay Multiple Lines 2"("Image"=w48, "Line End Points"=w60, "Drawing Mode (Frame)"=w75, "Color"=u32 16860, "Width"=u32 15) -> ("Image Out"=→"Image 7":T2)  [unwired: 9 in, 1 out]
        n62 = Subtract(x=w37, y=w36) -> (x-y=w35:i32)
        n63 = Divide(x=w35, y=2) -> (x/y=→"长度":dbl)
        n64 = Or(x=w102, y="Stop") -> (x .or. y?=w92:bool)
        "时间" <- w39
      }
    }
    frame #3 {
      # "4. The error -314220 indicates that the other endpoint has been destroyed. The VI ignores this error."
      # "3. Destroy the stream endpoint when you click Stop or when an error occurs."
      # "Close"
      n65 = Flush Stream(8:w247, 11:w250) -> (0:w248:errorcluster, 3:w249:refnum<k21>)  [unwired: 2 in, 1 out]
      n66 = Destroy Stream Endpoint(8:w248, 11:w249) -> (0:w242:errorcluster)
      n67 = Unbundle By Name(w242) -> ("code"=w246:i32)
      n68 = xnode "Error Ring"() -> ("错误输出"=w243:errorcluster)
      n69 = Not Equal?(x=w246, y=-314220) -> (x != y?=w244:bool)
      n70 = Select(t=w242, s=w244, f=w243) -> (s? t:f=→"error out":errorcluster)
    }
  }
